vi "Nivel_tanque.vi"() -> ()   [LabVIEW 2024]
panel:
  out "Numeric":dbl
  in  "Stop Button":bool
  in  "alpha":dbl min=0.0 max=1.0 step=0.05
  in  "Configuración válvula a1":T1(ring)
  in  "A":dbl=2.0 min=2.0 max=100.0 step=0.05
  in  "dt":dbl min=0.0 step=0.05
  in  "ht-1":dbl min=0.0 max=10.0 step=0.05
  in  "a2":dbl min=0.0 step=0.05
  in  "a1":dbl min=0.0 max=1.0 step=0.1
  in  "k2":dbl min=0.0 step=0.05
  out "ht":dbl(slide) scale=0.0..10.0
  in  "k1":dbl min=0.0 step=0.05
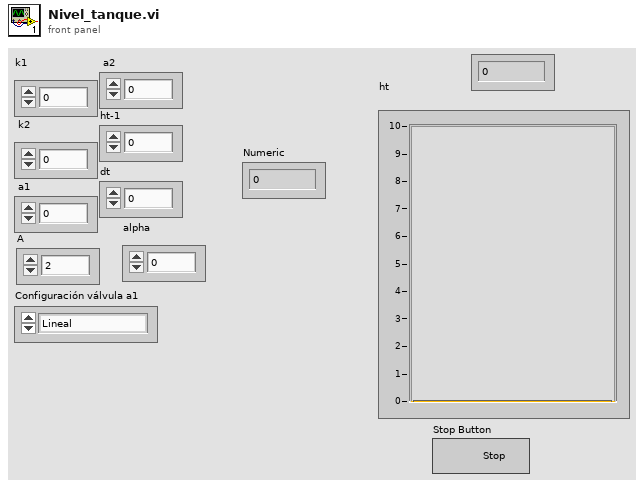
[diagram p1: front panel]
types:
  T1 = enum16{"Lineal", "Isopercentual", "Apertura rápida"}
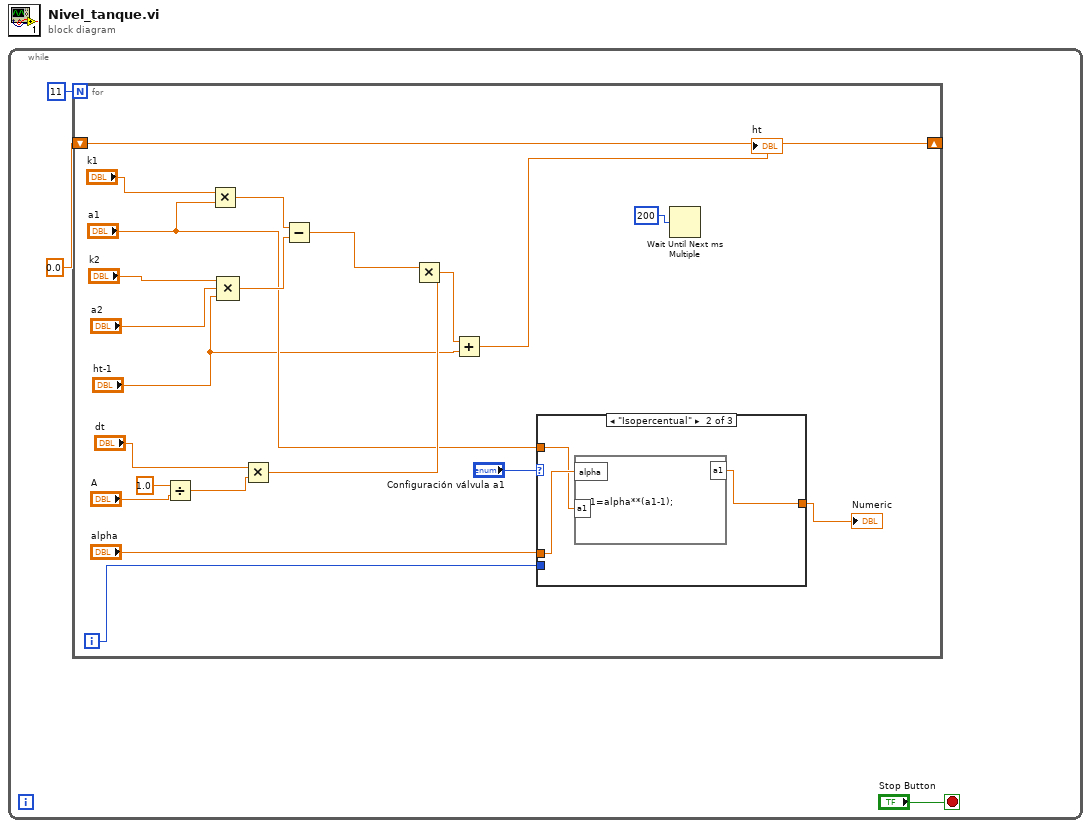
[diagram p0: block diagram]
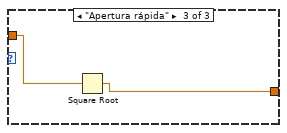
[diagram p3: hidden frame]
diagram:
  n1 = while {
    stop <- "Stop Button" stop-if-true
    n2 = for {
      N: 11 -> [_]
      shift-right: [w4] -> _
      shift-left: 0.0 -> [w4]
      i -> [w7]
      n3 = Divide(x=1.0, y="A") -> (x/y=w16:dbl)
      n4 = Multiply(x="k1", y="a1") -> (x*y=w21:dbl)
      n5 = Compound Arithmetic op=MULTIPLY("k2", "a2", "ht-1") -> (w20:dbl)
      n6 = Multiply(x="dt", y=w16) -> (x*y=w15:dbl)
      n7 = Subtract(x=w21, y=w20) -> (x-y=w14:dbl)
      n8 = Multiply(x=w14, y=w15) -> (x*y=w13:dbl)
      n9 = Add(x=w13, y="ht-1") -> (x+y=→"ht":dbl)
      n10 = case shown="\"Isopercentual\"" "Configuración válvula a1" {
        tunnel: "a1" -> [w25 w27 w30]
        tunnel: "alpha" -> [_ w28 _]
        tunnel: [w25 w26 w29] -> w8
        tunnel: w7 -> [_ _ _]
        frame "Lineal", Default {
        }
        frame "Isopercentual" {
          n11 = formula code="a1=alpha**(a1-1);"("alpha"=w28, "a1"=w27) -> ("a1"=w26:dbl)
        }
        frame "Apertura rápida" {
          n12 = Square Root(x=w30) -> (sqrt(x)=w29:dbl)
        }
      }
      "Numeric" <- w8
      n13 = Wait Until Next ms Multiple(millisecond multiple=u32 200) -> ()  [unwired: 1 out]
    }
  }
